vi "Configure ECU PWM Shifter.vi"(8 "error in (no error)":errorcluster, 9 "NIVS.System Definition Root":refnum<k24>, 10 "VI Reference":refnum<vi>, 11 "FNR Data in":T1) -> (0 "error out":errorcluster, 3 "FNR Data Out":T1)   [LabVIEW 2013]
doc: "Use this template to create a dialog box with event handling."
uses:
  NationalInstruments.VeriStand.SystemStorage
  Support/FNR Object Parameters.ctl
  Support/PWM Object Parameters.ctl
  <vilib>/NI Veristand/UI Controls/Single Node Browser/NI_VS UI Single Node Browser.lvlib
  NationalInstruments.VeriStand.SystemStorageUI
panel:
  in  "Make Current Values Default":bool
  in  "Reverse PWM":dbl=0.3 min=0.0 max=1.0 step=0.0001
  in  "Neutral PWM":dbl=0.2 min=0.0 max=1.0 step=0.0001
  in  "Forward PWM":dbl=0.8 min=0.0 max=1.0 step=0.0001
  in  "BG color":u32(colorbox)=16777228
  in  "Control Color":u32(colorbox)=16761088
  in  "RIO?":bool caption="Hardware type - click to toggle"
  in  "Control Label":string
  out "PWM Config Tab":enum32{"DAQ", "RIO"}(tab)
  in  "OK":bool
  in  "Cancel":bool
  in  "Selected Channel":refnum<k24>(container)
  # "PWM Duty Cycle"
  # "DAQ\nPWM\nRatio"
  # "FPGA\nPWM\n%"
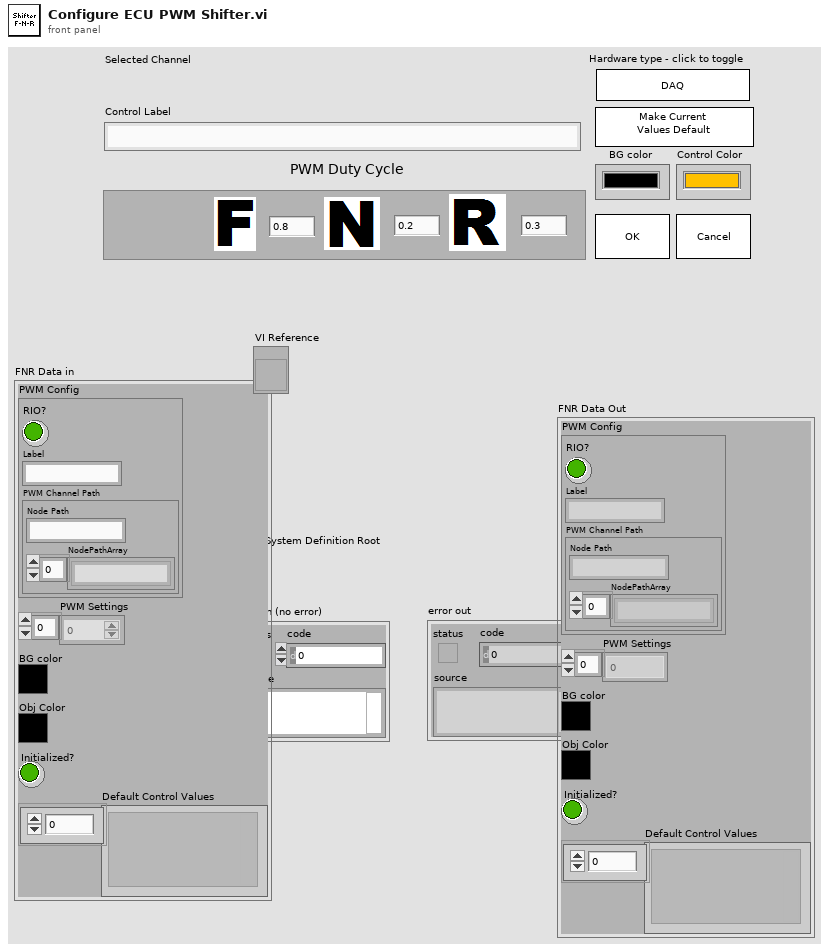
[diagram p1: front panel]
types:
  T1 = typedef "FNR Object Parameters.ctl" = cluster{"PWM Config":T2, "PWM Settings":dbl[], "BG color":u32, "Obj Color":u32, "Initialized?":bool, "Default Control Values":variant[]}
  T2 = typedef "PWM Object Parameters.ctl" = cluster{"RIO?":bool, "Label":string, "PWM Channel Path":cluster{"NodePathArray":string[], "Node Path":string}}
  T3 = typedef "NI_VS UI Single Node Browser.lvlib/Callback Type.ctl" = cluster{"Net Callbacks":refnum<k27>[], "Event":refnum<user-event>}
  T4 = typedef "NI_VS UI Single Node Browser.lvlib/Node Ref.ctl" = refnum<k24>
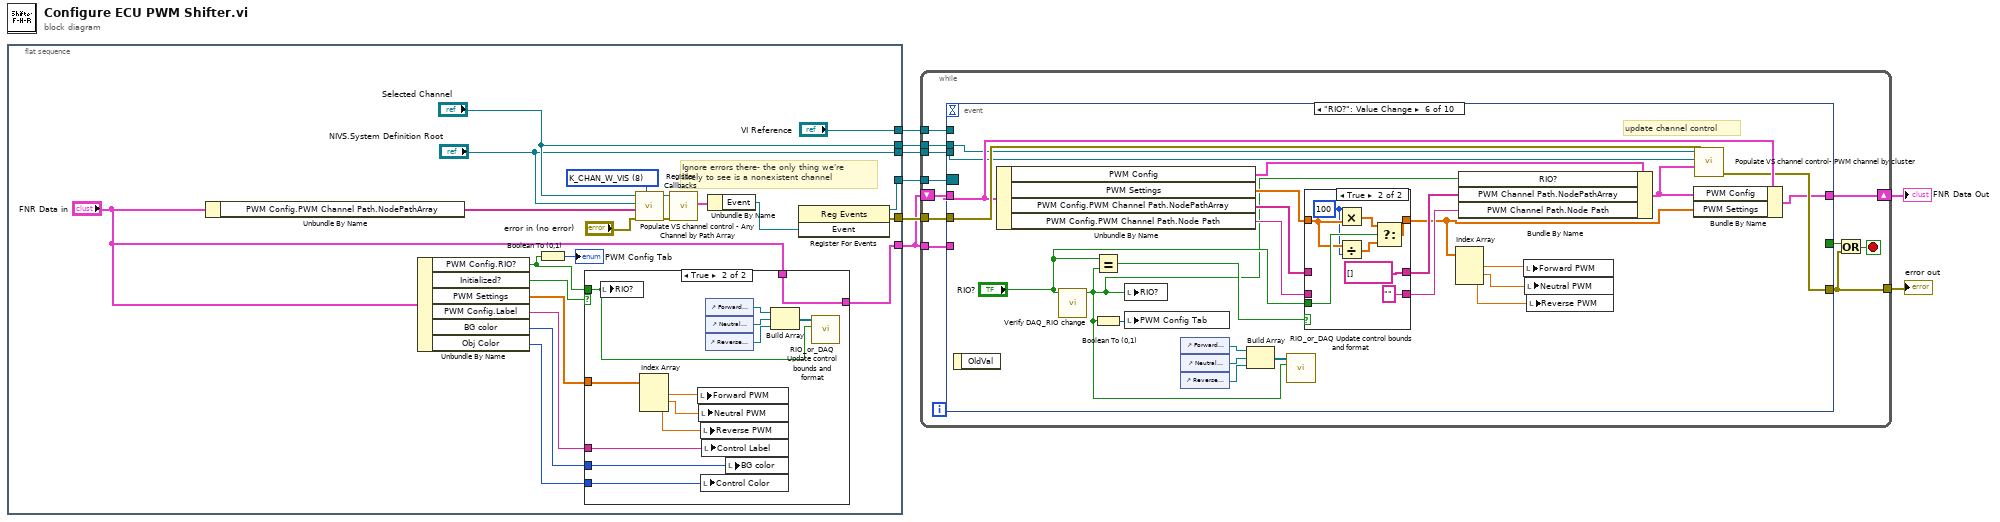
[diagram p0: block diagram]
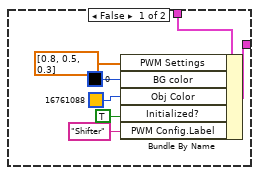
[diagram p2: hidden frame]
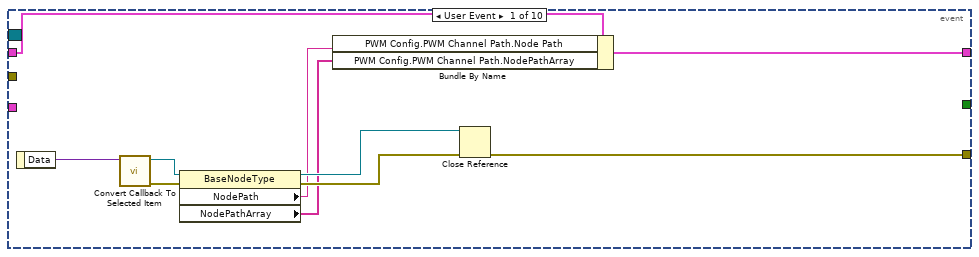
[diagram p3: hidden frame]
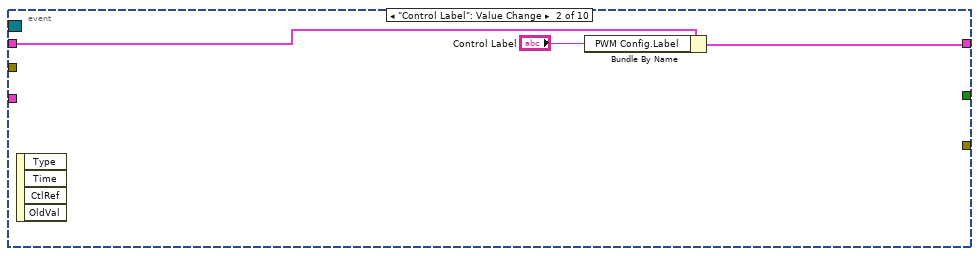
[diagram p4: hidden frame]
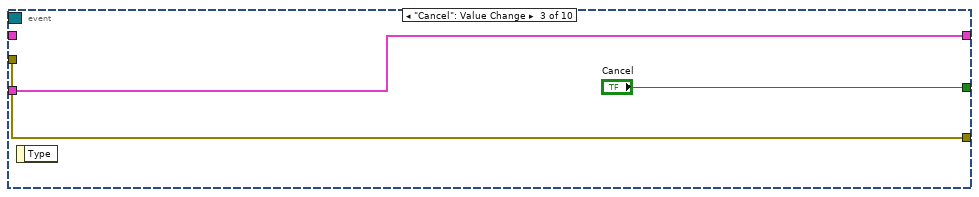
[diagram p5: hidden frame]
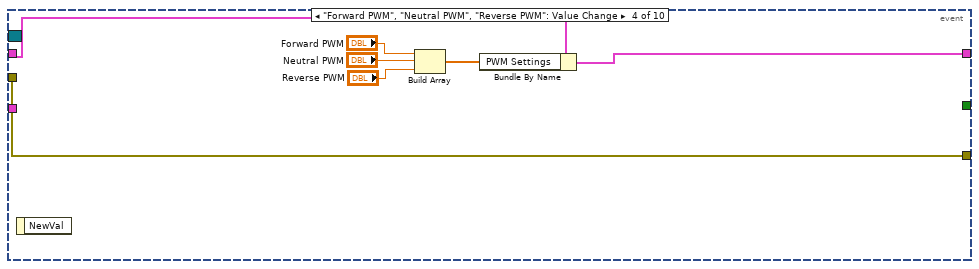
[diagram p6: hidden frame]
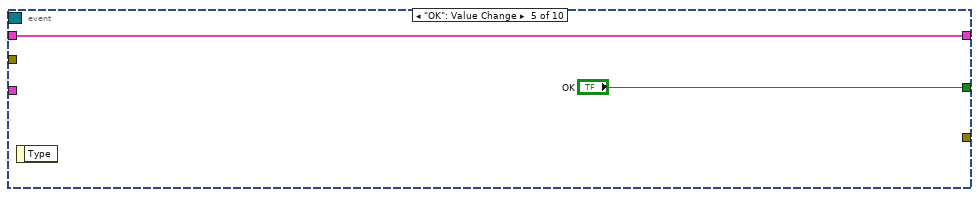
[diagram p7: hidden frame]
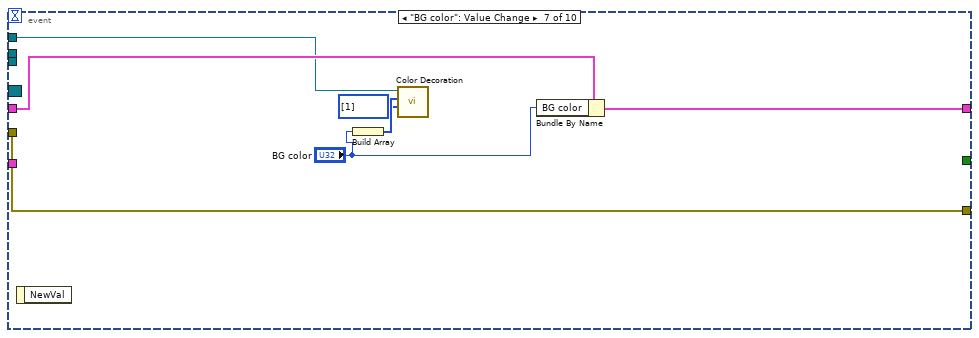
[diagram p9: hidden frame]
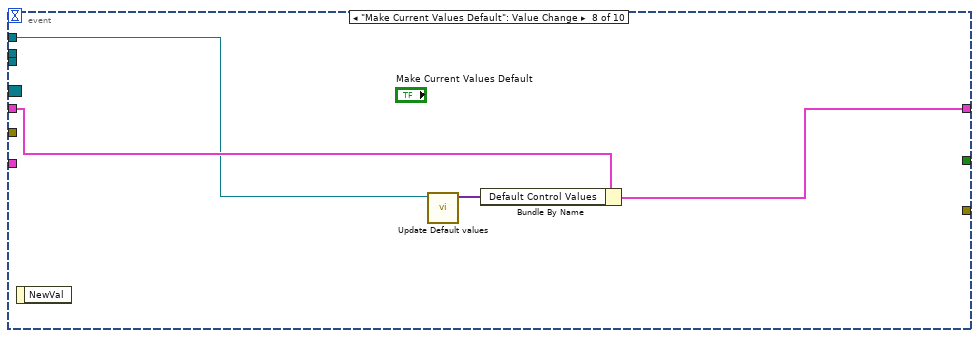
[diagram p10: hidden frame]
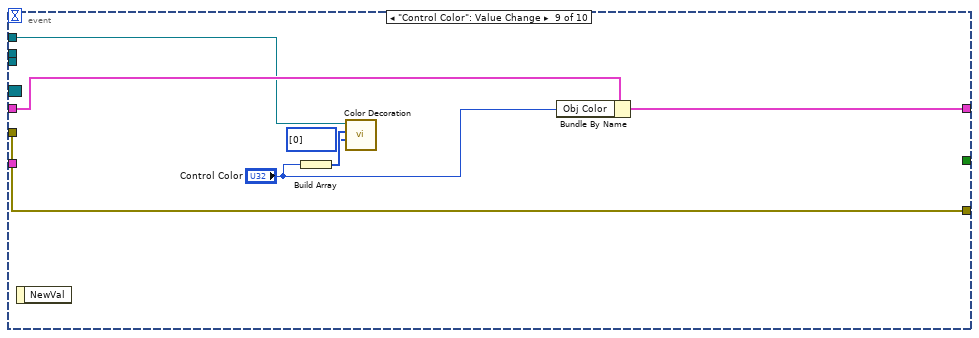
[diagram p11: hidden frame]
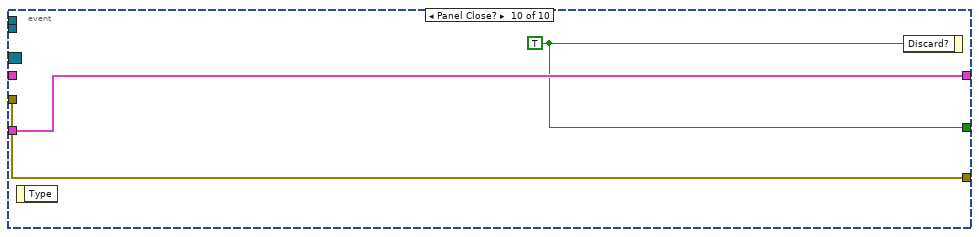
[diagram p12: hidden frame]
diagram:
  n1 = flat-sequence {
    tunnel: ["Selected Channel"] -> w7
    tunnel: ["NIVS.System Definition Root"] -> w6
    tunnel: [w13] -> w5
    tunnel: [w19] -> w3
    tunnel: ["VI Reference"] -> w2
    tunnel: [w12] -> w1
    frame #0 {
      w28 = u8 8 items=["K_CHAN_R", "K_CHAN_W", "K_CHAN_RW", "K_CHAN_VOLT", "K_CHAN_FAULT", "K_ALL", "K_CUSTOM", "K_CHAN_R_VIS", "K_CHAN_W_VIS", "K_CHAN_RW_VIS", "K_CHAN_VOLT_VIS", "K_CHAN_FAULT_VIS"] ("DisplayFilter")
      # "Ignore errors there- the only thing we're\nlikely to see is a nonexistent channel"
      n2 = Unbundle By Name("FNR Data in") -> ("PWM Config.PWM Channel Path.NodePathArray"=w9:string[])
      n3 = Unbundle By Name("FNR Data in") -> ("PWM Config.RIO?"=w11:bool, "Initialized?"=w21:bool, "PWM Settings"=w25:dbl[], "PWM Config.Label"=w24:string, "BG color"=w23:u32, "Obj Color"=w22:u32)
      n4 = Boolean To (0,1)(Boolean=w11) -> (0, 1=→"PWM Config Tab":i16)
      n5 = case shown="True" w21 {
        tunnel: w25 -> [_ w46]
        tunnel: w24 -> [_ w45]
        tunnel: w23 -> [_ w44]
        tunnel: w22 -> [_ w43]
        tunnel: "FNR Data in" -> [w36 w42]
        tunnel: [w35 w42] -> w19
        tunnel: w11 -> [_ w37]
        frame False {
          n6 = Bundle By Name(cluster=w36, "PWM Settings"=dbl[] [0.8, 0.5, 0.3] ("RIO PWM Settings"), "BG color"=u32 0, "Obj Color"=u32 16761088, "Initialized?"=TRUE ("New?"), "PWM Config.Label"="Shifter" ("Label")) -> (w35:T1)
        }
        frame True {
          n7 = local write "RIO?"(w37) -> ()
          n8 = Index Array(array=w46) -> (element #1=w49:dbl, element #2=w48:dbl, element #3=w47:dbl)  [unwired: 3 in]
          n9 = local write "Forward PWM"(w49) -> ()
          n10 = local write "Neutral PWM"(w48) -> ()
          n11 = local write "Reverse PWM"(w47) -> ()
          n12 = local write "Control Color"(w43) -> ()
          n13 = local write "Control Label"(w45) -> ()
          n14 = control-ref of="Forward PWM"() -> (w39:refnum<vi>)
          n15 = control-ref of="Neutral PWM"() -> (w40:refnum<vi>)
          n16 = control-ref of="Reverse PWM"() -> (w41:refnum<vi>)
          n17 = local write "BG color"(w44) -> ()
          n18 = Build Array(w39, w40, w41) -> (w38:refnum<vi>[])
          n19 = call "RIO_or_DAQ Update control bounds and format.vi"("RIO? in"=w37, "Control References in"=w38) -> ()  [unwired: 10 in]
        }
      }
      n20 = call "Populate VS channel control - Any Channel by Path Array.vi"("DisplayFilter"=w28, "error in (no error)"="error in (no error)", "Path Array In"=w9, "NIVS.System Definition Root"="NIVS.System Definition Root", ".NET Refnum in"="Selected Channel") -> ("error out"=w14:errorcluster, ".NET Refnum out"=w15:refnum<k24>)  [unwired: 5 in]
      n21 = call <vilib>:"Register Callbacks.vi"("error in (no error)"=w14, "Single Node Browser"=w15) -> ("Callbacks"=w17:T3)  [unwired: 7 in, 2 out]
      n22 = Unbundle By Name(w17) -> ("Event"=w16:refnum<user-event>)
      n23 = register-events(w16) -> (reference out=w12:refnum<event-registration>, error out=w13:errorcluster)  [unwired: 2 in]
    }
  }
  n24 = while {
    tunnel: [w50] -> w8
    shift-right: [w57] -> w4
    shift-left: w3 -> [w59]
    tunnel: w3 -> [w58]
    tunnel: w7 -> [w55]
    tunnel: w6 -> [w54]
    tunnel: w5 -> [w53]
    tunnel: w2 -> [w52]
    tunnel: w1 -> [w51]
    stop <- w56 stop-if-true
    n25 = event shown="[5] \"RIO?\": Value Change" {
      selector: w51 -> [_ _ _ _ _ _ _ _ _ _]
      dyn-events: _ -> [_ _ _ _ _ _ _ _ _ _]
      timeout: _ -> [_ _ _ _ _ _ _ _ _ _]
      tunnel: [_ _ "Cancel" _ "OK" _ _ _ _ w141] -> w60
      tunnel: [w62 _ w74 w83 _ w93 w126 _ w137 w140] -> w50
      tunnel: w59 -> [w63 w72 _ w82 w84 w96 w127 w131 w138 _]
      tunnel: w58 -> [_ _ w75 _ _ _ _ _ _ w142]
      tunnel: [w61 w73 w75 w81 w84 w92 w128 w130 w139 w142] -> w57
      tunnel: w55 -> [_ _ _ _ _ w94 _ _ _ _]
      tunnel: w54 -> [_ _ _ _ _ w95 _ _ _ _]
      tunnel: w53 -> [_ _ w74 w83 _ w97 w126 _ w137 w140]
      tunnel: w52 -> [_ _ _ _ _ _ w122 w129 w133 _]
      event User Event {
        n26 = event-data() -> ("Data"=w64:variant)  [unwired: 1 in]
        n27 = call <vilib>:"Convert Callback To Selected Item.vi"("Data"=w64) -> ("error out"=w67:errorcluster, "Selected Item"=w70:T4)  [unwired: 9 in]
        n28 = property class="BaseNodeType"(reference=w70, error in=w67) -> (reference out=w69:T4, error out=w68:errorcluster, "NodePath"=w66:string, "NodePathArray"=w65:string[])
        n29 = Bundle By Name(cluster=w63, "PWM Config.PWM Channel Path.Node Path"=w66, "PWM Config.PWM Channel Path.NodePathArray"=w65) -> (w61:T1)
        n30 = Close Reference(reference=w69, error in (no error)=w68) -> (error out=w62:errorcluster)
      }
      event "Control Label": Value Change {
        n31 = event-data() -> ()  [unwired: 1 in, 4 out]
        n32 = Bundle By Name(cluster=w72, "PWM Config.Label"="Control Label") -> (w73:T1)
      }
      event "Cancel": Value Change {
        n33 = event-data() -> ()  [unwired: 1 in, 1 out]
      }
      event "Forward PWM", "Neutral PWM", "Reverse PWM": Value Change {
        n34 = event-data() -> ()  [unwired: 1 in, 1 out]
        n35 = Build Array("Forward PWM", "Neutral PWM", "Reverse PWM") -> (w77:dbl[])
        n36 = Bundle By Name(cluster=w82, "PWM Settings"=w77) -> (w81:T1)
      }
      event "OK": Value Change {
        n37 = event-data() -> ()  [unwired: 1 in, 1 out]
      }
      event "RIO?": Value Change {
        # "update channel control"
        n38 = event-data() -> ()  [unwired: 1 in, 1 out]
        n39 = Unbundle By Name(w96) -> ("PWM Config"=w98:T2, "PWM Settings"=w100:dbl[], "PWM Config.PWM Channel Path.NodePathArray"=w101:string[], "PWM Config.PWM Channel Path.Node Path"=w102:string)
        n40 = call "Verify DAQ_RIO change.vi"("RIO? in"="RIO?") -> ("RIO? out"=w87:bool)  [unwired: 10 in]
        n41 = Equal?(x="RIO?", y=w87) -> (x = y?=w103:bool)
        n42 = Boolean To (0,1)(Boolean=w87) -> (0, 1=w106:i16)
        n43 = local write "RIO?"(w87) -> ()
        n44 = local write "PWM Config Tab"(w106) -> ()
        n45 = control-ref of="Forward PWM"() -> (w90:refnum<vi>)
        n46 = control-ref of="Neutral PWM"() -> (w89:refnum<vi>)
        n47 = control-ref of="Reverse PWM"() -> (w88:refnum<vi>)
        n48 = Build Array(w90, w89, w88) -> (w91:refnum<vi>[])
        n49 = call "RIO_or_DAQ Update control bounds and format.vi"("RIO? in"=w87, "Control References in"=w91) -> ()  [unwired: 10 in]
        n50 = case shown="True" w103 {
          tunnel: w100 -> [w113 w116]
          tunnel: "RIO?" -> [_ w120]
          tunnel: [w113 w119] -> w86
          tunnel: w101 -> [w112 _]
          tunnel: [w112 string[] [] ("NodePathArray")] -> w104
          tunnel: w102 -> [w111 _]
          tunnel: [w111 "" ("Node Path")] -> w105
          frame False {
          }
          frame True {
            w115 = 100
            n51 = Multiply(x=w115, y=w116) -> (x*y=w121:dbl[])
            n52 = Divide(x=w116, y=w115) -> (x/y=w118:dbl[])
            n53 = Select(t=w121, s=w120, f=w118) -> (s? t:f=w119:dbl[])
          }
        }
        n54 = Index Array(array=w86) -> (element #1=w110:dbl, element #2=w109:dbl, element #3=w108:dbl)  [unwired: 3 in]
        n55 = Bundle By Name(cluster=w98, "RIO?"=w87, "PWM Channel Path.NodePathArray"=w104, "PWM Channel Path.Node Path"=w105) -> (w99:T2)
        n56 = local write "Forward PWM"(w110) -> ()
        n57 = local write "Neutral PWM"(w109) -> ()
        n58 = local write "Reverse PWM"(w108) -> ()
        n59 = Bundle By Name(cluster=w96, "PWM Config"=w99, "PWM Settings"=w86) -> (w92:T1)
        n60 = call "Populate VS channel control- PWM channel by cluster.vi"("error in (no error)"=w97, "Data cluster in"=w99, "NIVS.System Definition Root"=w95, ".NET Refnum in"=w94) -> ("error out"=w93:errorcluster)  [unwired: 6 in, 1 out]
      }
      event "BG color": Value Change {
        n61 = event-data() -> ()  [unwired: 1 in, 1 out]
        n62 = Build Array("BG color") -> (w125:u32[])
        n63 = call "Color Decoration.vi"("VI reference"=w122, "Color Array"=w125, "Index Array"=u32[] [1]) -> ()  [unwired: 7 in, 1 out]
        n64 = Bundle By Name(cluster=w127, "BG color"="BG color") -> (w128:T1)
      }
      event "Make Current Values Default": Value Change {
        n65 = event-data() -> ()  [unwired: 1 in, 1 out]
        n66 = call "Update Default values.vi"("VI in"=w129) -> ("Default Values out"=w132:variant[])  [unwired: 10 in]
        n67 = Bundle By Name(cluster=w131, "Default Control Values"=w132) -> (w130:T1)
      }
      event "Control Color": Value Change {
        n68 = event-data() -> ()  [unwired: 1 in, 1 out]
        n69 = Build Array("Control Color") -> (w136:u32[])
        n70 = call "Color Decoration.vi"("VI reference"=w133, "Color Array"=w136, "Index Array"=u32[] [0]) -> ()  [unwired: 7 in, 1 out]
        n71 = Bundle By Name(cluster=w138, "Obj Color"="Control Color") -> (w139:T1)
      }
      event Panel Close? {
        w141 = TRUE ("Cancel")
        n72 = event-data() -> ()  [unwired: 1 in, 1 out]
        n73 = event-data("Discard?"=w141) -> ()  [unwired: 1 in, 1 out]
      }
    }
    n74 = Or(x=w60, y=w50) -> (x .or. y?=w56:bool)
  }
  "error out" <- w8
  "FNR Data Out" <- w4
